vi "Operation Data Status.vi"(6 "Operation Register Value To Set (0)":i32, 7 "Operation Register To Set (0: Enable)":i32(ring) items=["Enable", "NTR", "PTR"], 8 "error in (no error)":errorcluster, 9 "Operation Register To Check (0: Condition)":i32(ring) items=["Condition", "Enable", "Event", "NTR", "PTR"], 10 "Operation Mode (0: Check)":i32(ring) items=["Check", "Set"], 11 "VISA resource name":refnum<visa-resource-name>) -> (0 "error out":errorcluster, 2 "Operation Register Status":bool[](array[boolean]), 3 "VISA resource name out":refnum<visa-resource-name>)   [LabVIEW 2020, in "Agilent B2900 Series.lvlib"]
doc: "Sets or checks the Operation Data Status registers.\n\n<B>Note:</B> Use this VI only with other low-level VIs. The high-level VIs automatically incorporate this functionality. This VI does not check the instrument status."
uses:
  Agilent B2900 Series.lvlib
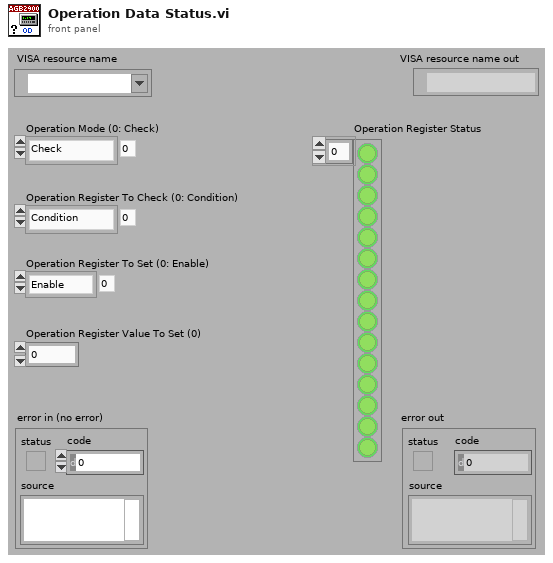
[diagram p1: front panel]
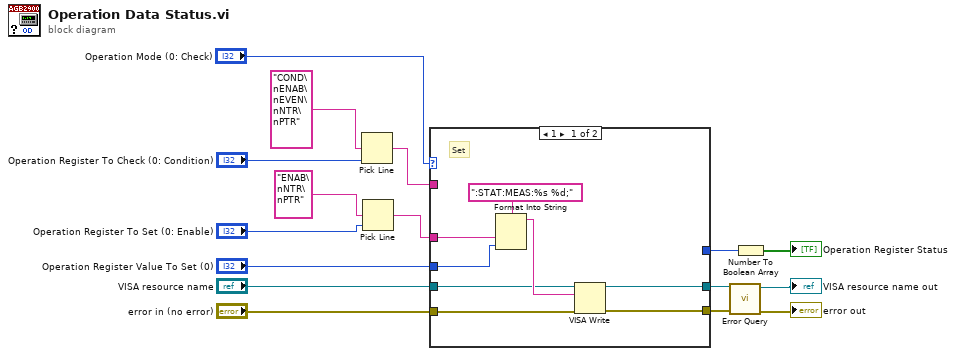
[diagram p0: block diagram]
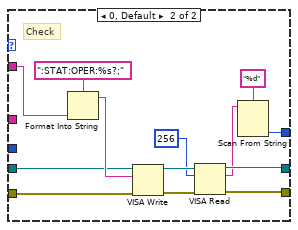
[diagram p2: hidden frame]
diagram:
  n1 = Pick Line(multi-line string="COND\nENAB\nEVEN\nNTR\nPTR", line index="Operation Register To Check (0: Condition)") -> (output string=w14:string)  [unwired: 1 in]
  n2 = Pick Line(multi-line string="ENAB\nNTR\nPTR", line index="Operation Register To Set (0: Enable)") -> (output string=w13:string)  [unwired: 1 in]
  n3 = case shown="1" "Operation Mode (0: Check)" {
    tunnel: w14 -> [_ w36]
    tunnel: [w21 w32] -> w1
    tunnel: [w20 w31] -> w2
    tunnel: [_ w27] -> w10
    tunnel: w13 -> [w24 _]
    tunnel: "VISA resource name" -> [w19 w26]
    tunnel: "error in (no error)" -> [w18 w25]
    tunnel: "Operation Register Value To Set (0)" -> [w17 _]
    frame 1 {
      # "Set"
      n4 = Format Into String(format string=":STAT:MEAS:%s %d;", w24, w17) -> (resulting string=w23:string)  [unwired: 2 in, 1 out]
      n5 = VISA Write(VISA resource name=w19, write buffer=w23, error in (no error)=w18) -> (VISA resource name out=w21:refnum<visa-resource-name>, error out=w20:errorcluster)  [unwired: 1 out]
    }
    frame 0, Default {
      # "Check"
      n6 = Format Into String(format string=":STAT:OPER:%s?;", w36) -> (resulting string=w35:string)  [unwired: 2 in, 1 out]
      n7 = VISA Write(VISA resource name=w26, write buffer=w35, error in (no error)=w25) -> (VISA resource name out=w33:refnum<visa-resource-name>, error out=w34:errorcluster)  [unwired: 1 out]
      n8 = VISA Read(VISA resource name=w33, byte count=u32 256, error in (no error)=w34) -> (VISA resource name out=w32:refnum<visa-resource-name>, read buffer=w29:string, error out=w31:errorcluster)  [unwired: 1 out]
      n9 = Scan From String(format string="%d", input string=w29) -> (output 1=w27:i32)  [unwired: 3 in, 3 out]
    }
  }
  n10 = call "Error Query.vi"("error in (no error)"=w2, "VISA resource name"=w1) -> ("error out"=→"error out":errorcluster, "VISA resource name out"=→"VISA resource name out":refnum<visa-resource-name>)  [unwired: 6 in, 2 out]
  n11 = Number To Boolean Array(number=w10) -> (Boolean array=→"Operation Register Status":bool[])
